vi "Start WiFi with DHCP.vi"(7 "Retry wait time [ms]":u32=2000, 8 "Error In":errorcluster, 11 "LINX Resource":T2) -> (0 "error out":errorcluster, 2 "TCP Configuration Out":T1, 3 "LINX Resource Out":T2={"IO"=enum."Remote", "Interface"=enum."Serial", "LINX Device Config"={"Interface"=enum."Serial", "COM Port"="COM13", "TCP Configuration"={"IP Address"="", "Port"=0}, "Device Family"=1, "Device ID"=1, "Device Name"="myRIO-1900", "TCP Ref"=refnum, "Channels"={"DI"=[0, 1, 2, 3, 4, 5, 6, 7, 8, 9, 10, 11, 12, 13, 14, 15, 16, 17, 18, 19, 20, 21, 22, 23, 24, 25, 26, 27, 28, 29, 30, 31, 32, 33, 34, 35, 36, 37, 38, 39, 40, 41, 42, 43, 44, 45, 46], "DO"=[0, 1, 2, 3, 4, 5, 6, 7, 8, 9, 10, 11, 12, 13, 14, 15, 16, 17, 18, 19, 20, 21, 22, 23, 24, 25, 26, 27, 28, 29, 30, 31, 32, 33, 34, 35, 36, 37, 38, 39, 40, 41, 42, 43, 44, 45, 46], "AI"=[0, 1, 2, 3, 4, 5, 6, 7, 8, 9, 10, 11], "AO"=[], "PWM"=[3, 5, 6, 9, 10], "QE"=[], "UART"=[0, 1], "I2C 2"=[0], "SPI"=[0], "CAN"=[], "Servo"=[], "AI Ref (V)"=0.0, "AI Resolution (Bits)"=0, "AO Ref (V)"=0.0, "AO Resolution (Bits)"=0}}})   [LabVIEW 2019, in "LINXx.lvlib"]
doc: "Attempts to connect board to network with DHCP. Returns dynamically-assigned IP if successful"
uses:
  LINXx.lvlib
  <vilib>/MakerHub/LINX/Private/Type Defs/LINX Ref.ctl
  <vilib>/MakerHub/LINX/Private/Type Defs/Platform.ctl
  <vilib>/MakerHub/LINX/Private/Type Defs/Interface.ctl
  <vilib>/MakerHub/LINX/Private/Device/Type Defs/LINX Device Config.ctl
  <vilib>/MakerHub/LINX/Private/Device/Type Defs/TCP Config.ctl
  <vilib>/MakerHub/LINX/Private/Device/Type Defs/Channels.ctl
  <vilib>/Utility/error.llb/Error Cluster From Error Code.vi
  <vilib>/ErrorRing/Error Ring.xnode
  <vilib>/MakerHub/LINX/Private/Device/Device.lvlib
  <vilib>/MakerHub/LINX/LMH-LINX.lvlib
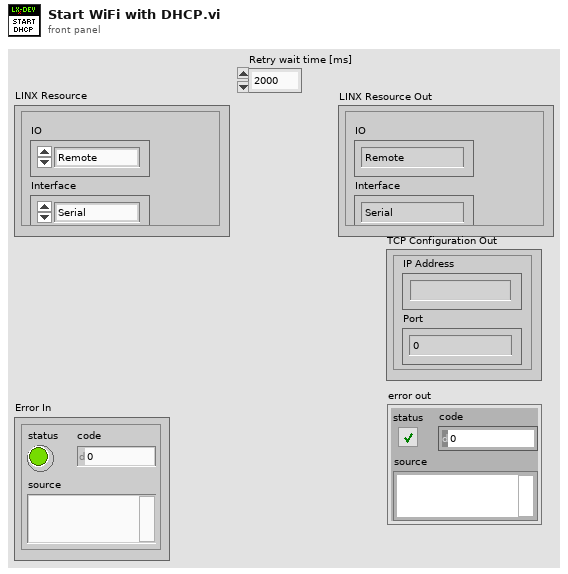
[diagram p1: front panel]
types:
  T1 = typedef "LMH-LINX.lvlib/Device.lvlib/TCP Config.ctl" = cluster{"IP Address":string, "Port":u16}
  T2 = typedef "LMH-LINX.lvlib/LINX Ref.ctl" = cluster{"IO":T3, "Interface":T4, "LINX Device Config":T5}
  T3 = typedef "LMH-LINX.lvlib/Platform.ctl" = enum16{"Remote", "Local"}
  T4 = typedef "LMH-LINX.lvlib/Interface.ctl" = enum16{"Serial", "TCP"}
  T5 = typedef "LMH-LINX.lvlib/Device.lvlib/LINX Device Config.ctl" = cluster{"Interface":T4, "COM Port":refnum<visa-resource-name>, "TCP Configuration":T1, "Device Family":u8, "Device ID":u8, "Device Name":string, "TCP Ref":refnum<k5>, "Channels":T6}
  T6 = typedef "LMH-LINX.lvlib/Channels.ctl" = cluster{"DI":u8[], "DO":u8[], "AI":u8[], "AO":u8[], "PWM":u8[], "QE":u8[], "UART":u8[], "I2C 2":u8[], "SPI":u8[], "CAN":u8[], "Servo":u8[], "AI Ref (V)":dbl, "AI Resolution (Bits)":u8, "AO Ref (V)":dbl, "AO Resolution (Bits)":u8}
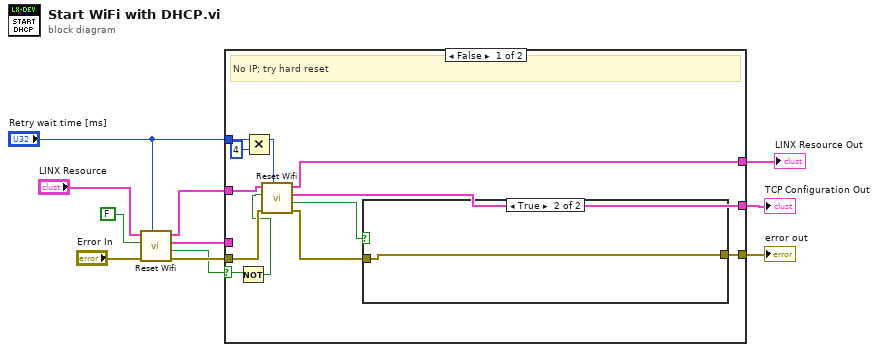
[diagram p0: block diagram]
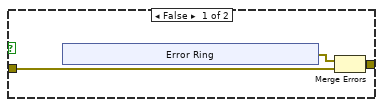
[diagram p2: hidden frame]
diagram:
  n1 = call "Reset Wifi.vi"("Retry wait time [ms]"="Retry wait time [ms]", "error in (no error)"="Error In", "Hard Reset?"=FALSE, "LINX Resource"="LINX Resource") -> ("error out"=w11:errorcluster, "Connected?"=w4:bool, "TCP Config"=w3:T1, "LINX Resource Out"=w6:T2)  [unwired: 4 in]
  n2 = case shown="False" w4 {
    selector: w4 -> [w17 _]
    tunnel: w11 -> [w20 w35]
    tunnel: [w23 w35] -> w9
    tunnel: w6 -> [w22 w34]
    tunnel: [w19 w34] -> w5
    tunnel: [w18 w33] -> w2
    tunnel: w3 -> [_ w33]
    tunnel: "Retry wait time [ms]" -> [w15 _]
    frame False {
      # "No IP; try hard reset"
      n3 = Not(x=w17) -> (.not. x?=w16:bool)
      n4 = Multiply(x=w15, y=u32 4) -> (x*y=w13:u32)
      n5 = call "Reset Wifi.vi"("Retry wait time [ms]"=w13, "error in (no error)"=w20, "Hard Reset?"=w16, "LINX Resource"=w22) -> ("error out"=w21:errorcluster, "Connected?"=w14:bool, "TCP Config"=w18:T1, "LINX Resource Out"=w19:T2)  [unwired: 4 in]
      n6 = case shown="True" w14 {
        tunnel: [w25 w32] -> w23
        tunnel: w21 -> [w24 w32]
        frame False {
          n7 = xnode "Error Ring"() -> ("error out"=w26:errorcluster)
          n8 = Merge Errors(w26, w24) -> (w25:errorcluster)
        }
        frame True {
        }
      }
    }
    frame True {
      # "Success, got new IP"
    }
  }
  "LINX Resource Out" <- w5
  "TCP Configuration Out" <- w2
  "error out" <- w9
